vi "AK Auswerten.vi"(10 "Array":string[](array[string])) -> ()   [LabVIEW 2020, in "FT-IR.lvlib" / "AK-Interface.lvlib"]
uses:
  AK-Interface.lvlib
  FGV FT-IR Aktionen.ctl
  Aktionen EVID-Codes.ctl
  Status Analysatoren/Aktion Status Analysatoren.ctl
  Messdaten/Aktionen FGV Messwerte zusammenfassen.ctl
  System Einstellungen V2/Aktioen FGV System.ctl
  Messdaten/Aktionen FGV Messdaten logging.ctl
  Span/Aktion FGV Span.ctl
  Span/Aktion FGV SGSF und SGSO weiterleiten.ctl
  Log Konfig/Aktion LabBaseIndex.ctl
  Messdaten/Messdaten.lvlib
  FT-IR.lvlib
  Status Analysatoren/Status Analysatoren.lvlib
  System Einstellungen V2/System Einstellungen V2.lvlib
  Log Konfig/LogKonfig.lvlib
  Span/Spanfaktor.lvlib
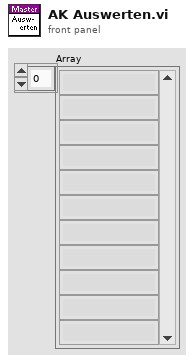
[diagram p1: front panel]
types:
  T1 = typedef "Messdaten.lvlib/Aktionen FGV Messwerte zusammenfassen.ctl" = enum16{"lesen", "FT-IR", "Algebraic", "LabBaseName", "LabBaseNr"}
  T2 = typedef "System Einstellungen V2.lvlib/Aktioen FGV System.ctl" = enum16{"lesen", "laden", "speichern", "Optionen schreiben", "Zeitstempel", "Reset BMP", "Reset SQP", "Wartung", "Werkseinstellung"}
  T3 = typedef "Status Analysatoren.lvlib/Aktion Status Analysatoren.ctl" = enum16{"lesen", "initialisieren", "Analysatoren aktiv", "FTIR Fehler", "FID Fehler", "PMA Fehler", "Felder einfärben"}
  T4 = typedef "FT-IR.lvlib/Aktionen EVID-Codes.ctl" = enum16{"lesen", "setzen", "laden", "speichern", "1Hz/5Hz", "Smoothing", "Rolling Average"}
  T5 = typedef "FT-IR.lvlib/FGV FT-IR Aktionen.ctl" = enum16{"lesen", "NOG setzen", "NOS setzen", "Initialisieren", "speichern", "ALLES setzen", "FT-IR Spektrum loggen", "Komm Stoppen", "Spektrum LogKonfig"}
  T6 = typedef "Messdaten.lvlib/Aktionen FGV Messdaten logging.ctl" = enum16{"lesen", "schreiben", "init", "löschen", "werte eintakten", "Flag setzen"}
  T7 = cluster{"Neue Messwerte":sgl[], "Labbase Name+Nr":string}
  T8 = typedef "FT-IR.lvlib/Spanfaktor.lvlib/Aktion FGV SGSF und SGSO weiterleiten.ctl" = enum16{"lesen", "AGSF", "AGSO", "AGSF löschen", "AGSO löschen", "SGSF", "SGSO", "SGSF löschen", "SGSO löschen"}
  T9 = typedef "FT-IR.lvlib/Spanfaktor.lvlib/Aktion FGV Span.ctl" = enum16{"lesen", "Span", "Seite aktiv", "Offset", "FGV aktualisiert", "Aktualisierung aufheben"}
  T10 = typedef "LogKonfig.lvlib/Aktion LabBaseIndex.ctl" = enum16{"lesen", "schreiben"}
  T11 = typedef "System Einstellungen V2.lvlib/Optionen.ctl" = cluster{"Störmeldep.":bool, "Betriebszustände":bool, "AK in ppm":bool, "log Cal-Gas":bool, "log 0-Gas":bool, "Durchflusssensor 0-5V":bool, "PNS?":bool, "Mit N2 spülen":bool, "TRE08":bool, "Amium 10-Fach":bool, "Verticale Scrollbar aktiv":bool, "Loggingtakt":bool, "AK Rezeptwechsel gleich wie MKS":bool, "NG ECO":bool}
  T12 = cluster{"(80) labEnabled":bool, "(81) labPath":path, "(82) labBaseName":string, "(83) labIndex":string, "Spektrum loggen aktiv?":bool}
  T13 = typedef "Status Analysatoren.lvlib/Status.ctl" = cluster{"FT-IR aktiv":bool, "FT-IR Fehler":bool, "FID aktiv":bool, "FID Fehler":bool, "PMA aktiv":bool, "PMA Fehler":bool}
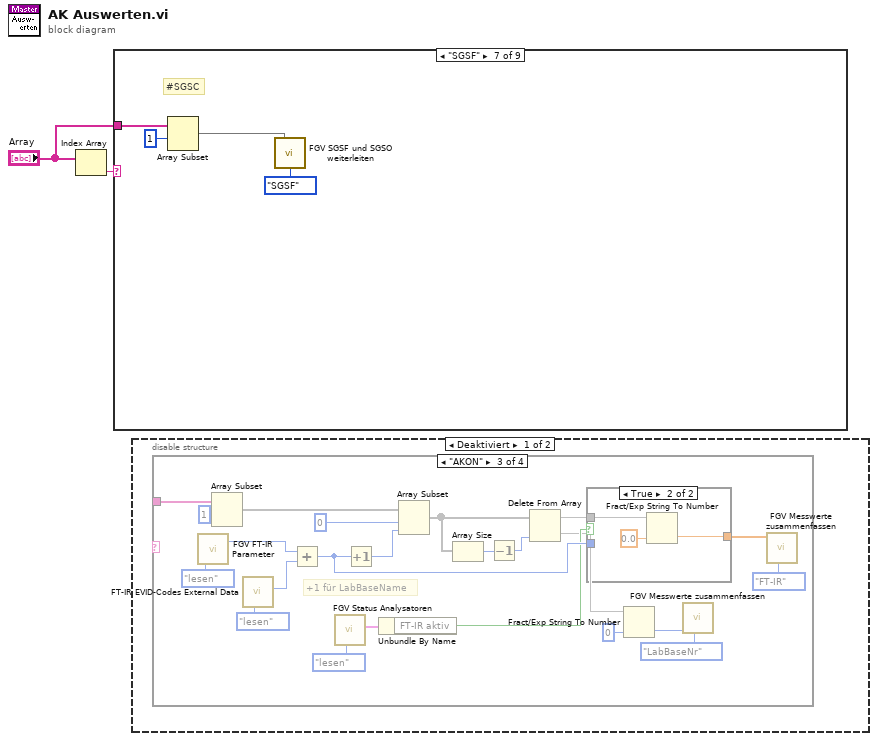
[diagram p0: block diagram]
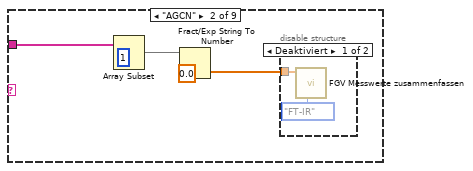
[diagram p3: hidden frame]
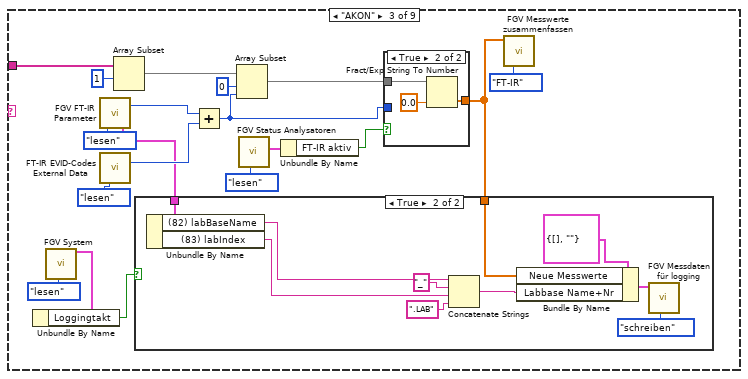
[diagram p5: hidden frame]
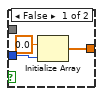
[diagram p7: hidden frame]
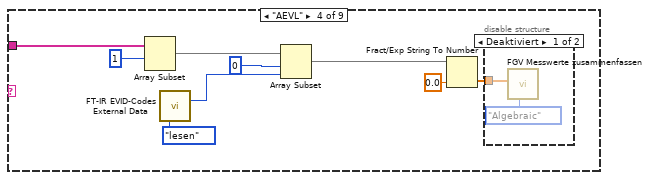
[diagram p8: hidden frame]
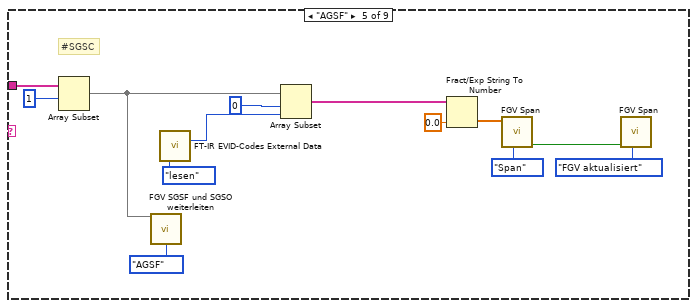
[diagram p10: hidden frame]
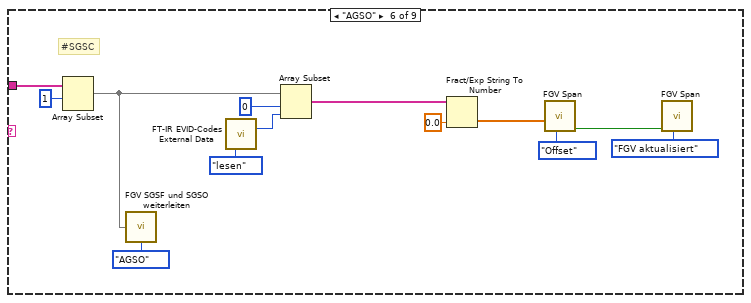
[diagram p11: hidden frame]
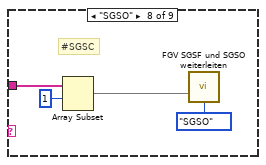
[diagram p12: hidden frame]
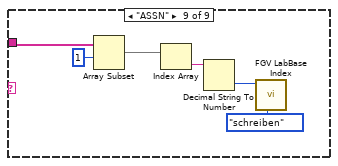
[diagram p13: hidden frame]
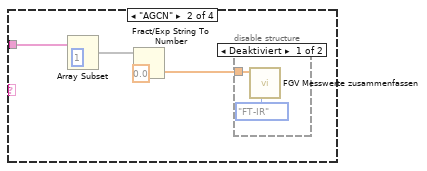
[diagram p15: hidden frame]
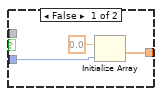
[diagram p17: hidden frame]
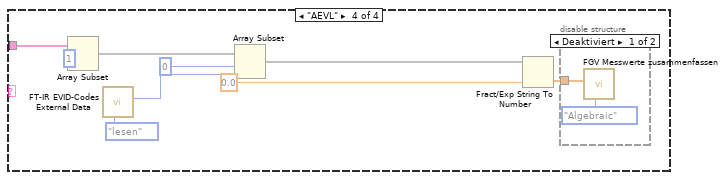
[diagram p18: hidden frame]
diagram:
  n1 = Index Array(array="Array") -> (element=w2:string)  [unwired: 1 in]
  n2 = case shown="\"SGSF\"" w2 {
    tunnel: "Array" -> [_ w7 w18 w53 w68 w70 w83 w87 w92]
    frame "False", Default {
    }
    frame "AGCN" {
      n3 = Array Subset(array=w7, index=1 ("Index")) -> (w5:string[])  [unwired: 1 in]
      n4 = Fract/Exp String To Number(string=w5, default (0 dbl)=sgl 0.0 ("Standard (0 DBL)")) -> (number=w3:sgl[])  [unwired: 2 in, 1 out]
      n5 = disable-structure shown="Deaktiviert" {
        disable-tunnel: w3 -> [w8 _]
        frame Disabled {
          n6 = call "FGV Messwerte zusammenfassen.vi"("Aktionen"=Aktionen_FGV_Messwerte_zusammenfassen."FT-IR", "FT-IR"=w8) -> ()  [unwired: 5 in, 5 out]
        }
        frame Enabled {
        }
      }
    }
    frame "AKON" {
      n7 = call "FGV System.vi"("Aktionen"=Aktioen_FGV_System."lesen") -> ("Optionen"=w11:T11)  [unwired: 12 in, 6 out]
      n8 = Unbundle By Name(w11) -> ("Loggingtakt"=w12:bool)
      n9 = call "FGV FT-IR Parameter.vi"("Aktion"=FGV_FT-IR_Aktionen."lesen") -> ("Ausgangs-Cluster"=w10:T12, "NoOfGasses"=w23:u32)  [unwired: 11 in, 6 out]
      n10 = call "FT-IR EVID-Codes External Data.vi"("Aktionen"=Aktionen_EVID-Codes."lesen") -> ("Anzahl"=w24:i32)  [unwired: 9 in, 5 out]
      n11 = Array Subset(array=w18, index=1 ("Index")) -> (w14:string[])  [unwired: 1 in]
      n12 = Add(x=w23, y=w24) -> (x+y=w20:u32)
      n13 = Array Subset(array=w14, index=0 ("Index"), length=w20) -> (w16:string[])
      n14 = call "FGV Status Analysatoren.vi"("Aktionen"=Aktion_Status_Analysatoren."lesen") -> ("Status Analysatoren"=w21:T13)  [unwired: 10 in]
      n15 = Unbundle By Name(w21) -> ("FT-IR aktiv"=w19:bool)
      n16 = case shown="True" w19 {
        tunnel: w16 -> [_ w43]
        tunnel: [w39 w42] -> w17
        tunnel: w20 -> [w40 _]
        frame False {
          n17 = Initialize Array(sgl 0.0 ("Element"), w40) -> (w39:sgl[])
        }
        frame True {
          n18 = Fract/Exp String To Number(string=w43, default (0 dbl)=sgl 0.0 ("Standard (0 DBL)")) -> (number=w42:sgl[])  [unwired: 2 in, 1 out]
        }
      }
      n19 = case shown="True" w12 {
        tunnel: w17 -> [_ w38]
        tunnel: w10 -> [_ w31]
        frame False {
        }
        frame True {
          n20 = Unbundle By Name(w31) -> ("(82) labBaseName"=w30:string, "(83) labIndex"=w29:string)
          n21 = Concatenate Strings(w30, "_" ("String"), w29, ".LAB" ("String")) -> (w35:string)
          n22 = Bundle By Name(cluster=T7 {"Neue Messwerte"=[], "Labbase Name+Nr"=""} ("AK Messwerte"), "Neue Messwerte"=w38, "Labbase Name+Nr"=w35) -> (w34:T7)
          n23 = call "FGV Messdaten für logging.vi"("Aktionen"=Aktionen_FGV_Messdaten_logging."schreiben", "AK Messwerte"=w34) -> ()  [unwired: 9 in, 1 out]
        }
      }
      n24 = call "FGV Messwerte zusammenfassen.vi"("Aktionen"=Aktionen_FGV_Messwerte_zusammenfassen."FT-IR", "FT-IR"=w17) -> ()  [unwired: 5 in, 5 out]
    }
    frame "AEVL" {
      n25 = Array Subset(array=w53, index=1 ("Index")) -> (w46:string[])  [unwired: 1 in]
      n26 = call "FT-IR EVID-Codes External Data.vi"("Aktionen"=Aktionen_EVID-Codes."lesen") -> ("Anzahl"=w47:i32)  [unwired: 9 in, 5 out]
      n27 = Array Subset(array=w46, index=0 ("Index"), length=w47) -> (w45:string[])
      n28 = Fract/Exp String To Number(string=w45, default (0 dbl)=sgl 0.0 ("Standard (0 DBL)")) -> (number=w50:sgl[])  [unwired: 2 in, 1 out]
      n29 = disable-structure shown="Deaktiviert" {
        disable-tunnel: w50 -> [w54 _]
        frame Disabled {
          n30 = call "FGV Messwerte zusammenfassen.vi"("Aktionen"=Aktionen_FGV_Messwerte_zusammenfassen."Algebraic", "Algebraic"=w54) -> ()  [unwired: 5 in, 5 out]
        }
        frame Enabled {
        }
      }
    }
    frame "AGSF" {
      # "#SGSC"
      n31 = Array Subset(array=w68, index=1 ("Index")) -> (w57:string[])  [unwired: 1 in]
      n32 = call "FGV SGSF und SGSO weiterleiten.vi"("AGSF"=w57, "Aktion"=Aktion_FGV_SGSF_und_SGSO_weiterleiten."AGSF") -> ()  [unwired: 5 in, 9 out]
      n33 = call "FT-IR EVID-Codes External Data.vi"("Aktionen"=Aktionen_EVID-Codes."lesen") -> ("Anzahl"=w63:i32)  [unwired: 9 in, 5 out]
      n34 = Array Subset(array=w57, index=0 ("Index"), length=w63) -> (w62:string[])
      n35 = Fract/Exp String To Number(string=w62, default (0 dbl)=sgl 0.0 ("Standard (0 DBL)")) -> (number=w60:sgl[])  [unwired: 2 in, 1 out]
      n36 = call "FGV Span.vi"("Aktion"=Aktion_FGV_Span."Span", "Span"=w60) -> ("Aktiv"=w58:bool)  [unwired: 6 in, 3 out]
      n37 = call "FGV Span.vi"("Aktion"=Aktion_FGV_Span."FGV aktualisiert", "Aktiv"=w58) -> ()  [unwired: 6 in, 4 out]
    }
    frame "AGSO" {
      # "#SGSC"
      n38 = Array Subset(array=w70, index=1 ("Index")) -> (w69:string[])  [unwired: 1 in]
      n39 = call "FGV SGSF und SGSO weiterleiten.vi"("AGSO"=w69, "Aktion"=Aktion_FGV_SGSF_und_SGSO_weiterleiten."AGSO") -> ()  [unwired: 5 in, 9 out]
      n40 = call "FT-IR EVID-Codes External Data.vi"("Aktionen"=Aktionen_EVID-Codes."lesen") -> ("Anzahl"=w77:i32)  [unwired: 9 in, 5 out]
      n41 = Array Subset(array=w69, index=0 ("Index"), length=w77) -> (w76:string[])
      n42 = Fract/Exp String To Number(string=w76, default (0 dbl)=sgl 0.0 ("Standard (0 DBL)")) -> (number=w75:sgl[])  [unwired: 2 in, 1 out]
      n43 = call "FGV Span.vi"("Aktion"=Aktion_FGV_Span."Offset", "Offset"=w75) -> ("Aktiv"=w72:bool)  [unwired: 6 in, 3 out]
      n44 = call "FGV Span.vi"("Aktion"=Aktion_FGV_Span."FGV aktualisiert", "Aktiv"=w72) -> ()  [unwired: 6 in, 4 out]
    }
    frame "SGSF" {
      # "#SGSC"
      n45 = Array Subset(array=w83, index=1 ("Index")) -> (w82:string[])  [unwired: 1 in]
      n46 = call "FGV SGSF und SGSO weiterleiten.vi"("SGSF"=w82, "Aktion"=Aktion_FGV_SGSF_und_SGSO_weiterleiten."SGSF") -> ()  [unwired: 5 in, 9 out]
    }
    frame "SGSO" {
      # "#SGSC"
      n47 = Array Subset(array=w87, index=1 ("Index")) -> (w86:string[])  [unwired: 1 in]
      n48 = call "FGV SGSF und SGSO weiterleiten.vi"("SGSO"=w86, "Aktion"=Aktion_FGV_SGSF_und_SGSO_weiterleiten."SGSO") -> ()  [unwired: 5 in, 9 out]
    }
    frame "ASSN" {
      n49 = Array Subset(array=w92, index=1 ("Index")) -> (w94:string[])  [unwired: 1 in]
      n50 = Index Array(array=w94) -> (element=w93:string)  [unwired: 1 in]
      n51 = Decimal String To Number(string=w93) -> (number=w90:i32)  [unwired: 2 in, 1 out]
      n52 = call "FGV LabBase Index.vi"("Aktion"=Aktion_LabBaseIndex."schreiben", "Index Nr. Start:"=w90) -> ()  [unwired: 8 in, 2 out]
    }
  }
  n53 = disable-structure shown="Deaktiviert" {
    frame Disabled {
      n54 = case shown="\"AKON\"" {
        selector: _ -> [_ _ _ _]
        tunnel: _ -> [_ w100 w125 w140]
        frame "False", Default {
        }
        frame "AGCN" {
          n55 = Array Subset(array=w100, index=1 ("Index")) -> (w98:void[])  [unwired: 1 in]
          n56 = Fract/Exp String To Number(string=w98, default (0 dbl)=sgl 0.0 ("Standard (0 DBL)")) -> (number=w96:sgl[])  [unwired: 2 in, 1 out]
          n57 = disable-structure shown="Deaktiviert" {
            disable-tunnel: w96 -> [w101 _]
            frame Disabled {
              n58 = call "FGV Messwerte zusammenfassen.vi"("Aktionen"=Aktionen_FGV_Messwerte_zusammenfassen."FT-IR", "FT-IR"=w101) -> ()  [unwired: 5 in, 5 out]
            }
            frame Enabled {
            }
          }
        }
        frame "AKON" {
          # "+1 für LabBaseName"
          n59 = call "FGV FT-IR Parameter.vi"("Aktion"=FGV_FT-IR_Aktionen."lesen") -> ("NoOfGasses"=w116:u32)  [unwired: 11 in, 7 out]
          n60 = Array Subset(array=w125, index=1 ("Index")) -> (w119:void[])  [unwired: 1 in]
          n61 = call "FT-IR EVID-Codes External Data.vi"("Aktionen"=Aktionen_EVID-Codes."lesen") -> ("Anzahl"=w118:i32)  [unwired: 6 in, 4 out]
          n62 = Add(x=w116, y=w118) -> (x+y=w112:u32)
          n63 = call "FGV Status Analysatoren.vi"("Aktionen"=Aktion_Status_Analysatoren."lesen") -> ("Status Analysatoren"=w113:T13)  [unwired: 10 in]
          n64 = Increment(x=w112) -> (x+1=w115:u32)
          n65 = Unbundle By Name(w113) -> ("FT-IR aktiv"=w111:bool)
          n66 = Array Subset(array=w119, index=0 ("Index"), length=w115) -> (w109:void[])
          n67 = Array Size(array=w109) -> (size(s)=w108:i32)
          n68 = Decrement(x=w108) -> (x-1=w107:i32)
          n69 = Delete From Array(array=w109, index=w107) -> (deleted portion=w105, array with subset deleted=w110)  [unwired: 1 in]
          n70 = case shown="True" w111 {
            tunnel: w110 -> [_ w130]
            tunnel: [w127 w129] -> w117
            tunnel: w112 -> [w126 _]
            frame False {
              n71 = Initialize Array(sgl 0.0 ("Element"), w126) -> (w127:sgl[])
            }
            frame True {
              n72 = Fract/Exp String To Number(string=w130, default (0 dbl)=sgl 0.0 ("Standard (0 DBL)")) -> (number=w129:sgl)  [unwired: 2 in, 1 out]
            }
          }
          n73 = Fract/Exp String To Number(string=w105, default (0 dbl)=0 ("Standard (0 DBL)")) -> (number=w103:i32)  [unwired: 2 in, 1 out]
          n74 = call "FGV Messwerte zusammenfassen.vi"("Aktionen"=Aktionen_FGV_Messwerte_zusammenfassen."LabBaseNr", "LabBaseNr"=w103) -> ()  [unwired: 5 in, 5 out]
          n75 = call "FGV Messwerte zusammenfassen.vi"("Aktionen"=Aktionen_FGV_Messwerte_zusammenfassen."FT-IR", "FT-IR"=w117) -> ()  [unwired: 5 in, 5 out]
        }
        frame "AEVL" {
          n76 = Array Subset(array=w140, index=1 ("Index")) -> (w133:void[])  [unwired: 1 in]
          n77 = call "FT-IR EVID-Codes External Data.vi"("Aktionen"=Aktionen_EVID-Codes."lesen") -> ("Anzahl"=w134:i32)  [unwired: 6 in, 4 out]
          n78 = Array Subset(array=w133, index=0 ("Index"), length=w134) -> (w132:void[])
          n79 = Fract/Exp String To Number(string=w132, default (0 dbl)=sgl 0.0 ("Standard (0 DBL)")) -> (number=w137:sgl[])  [unwired: 2 in, 1 out]
          n80 = disable-structure shown="Deaktiviert" {
            disable-tunnel: w137 -> [w141 _]
            frame Disabled {
              n81 = call "FGV Messwerte zusammenfassen.vi"("Aktionen"=Aktionen_FGV_Messwerte_zusammenfassen."Algebraic", "Algebraic"=w141) -> ()  [unwired: 5 in, 5 out]
            }
            frame Enabled {
            }
          }
        }
      }
    }
    frame Enabled {
    }
  }
